vi "About.vi"(0 "path":path) -> ()   [LabVIEW 2013]
uses:
  <vilib>/Platform/browser.llb/Open URL in Default Browser (string).vi
panel:
  out "Author:":string="Martin Šíra"
  out "E-mail:":string="msira@cmi.cz"
  in  "OK":bool
  out "address":string="Czech Metrology Institute\nDepartment of Primary Metrology of\nDC/LF Electrical Quantities\nOkružní 31\n63800, Brno\nCzech Republic"
  out "www:":string="https://qwtb.github.io/qwtb/"
  out "Version:":string
  # "simple QWTB GUI"
  # "Simple QWTB GUI is a front end to a QWTB with graphical user interface.\n\nQWTB is a toolbox for evaluation of measured data. QWTB consist of data processing algorithms from very different sources and unificating application interface. The toolbox gives the possibility to use different data processing algorithms with one set of data and removes the need to reformat data for every particular algorithm. Toolbox is extensible. The toolbox can variate input data and calculate uncertainties by means of Monte Carlo Method (MCM).\n\nToolbox was realized within the EMRP-Project SIB59\nQ-Wave. The EMRP is jointly funded by the EMRP par- ticipating countries within EURAMET and the European Union."
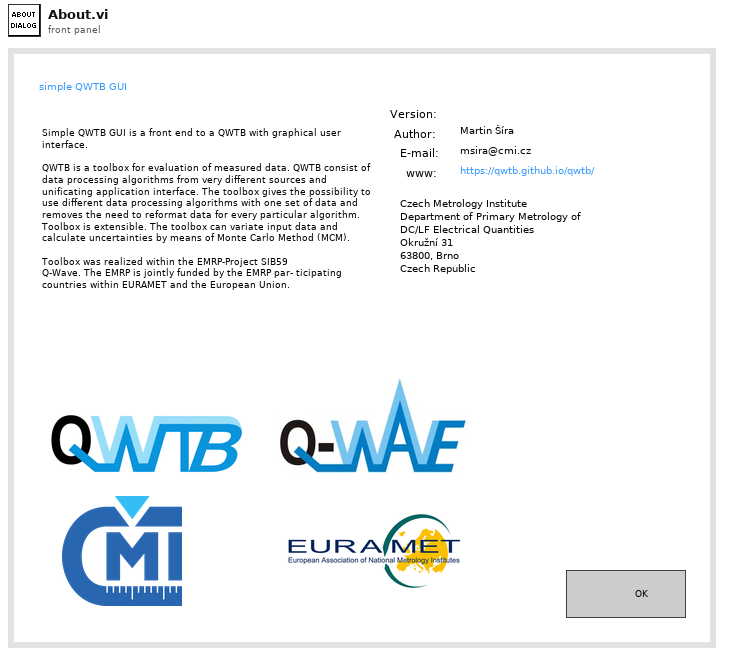
[diagram p1: front panel]
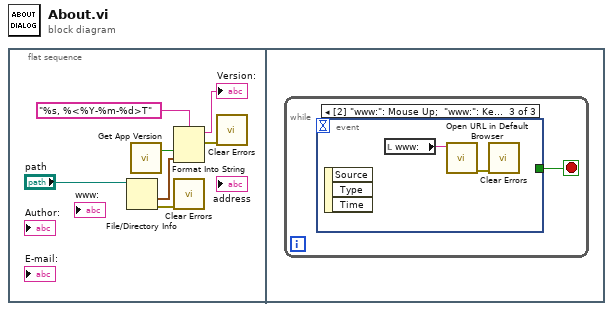
[diagram p0: block diagram]
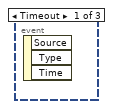
[diagram p2: hidden frame]
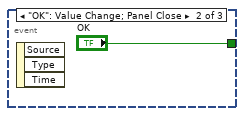
[diagram p3: hidden frame]
diagram:
  n1 = flat-sequence {
    frame #0 {
      n2 = File/Directory Info(path="path") -> (last mod=w4:timestamp, error out=w7:errorcluster)  [unwired: 1 in, 5 out]
      n3 = call "Get App Version.vi"() -> ("runtime"=w3:bool)  [unwired: 1 out]
      n4 = Format Into String(format string="%s, %<%Y-%m-%d>T" ("time format string (%c)"), w3, w4) -> (resulting string=→"Version:":string, error out=w5:errorcluster)  [unwired: 2 in]
      n5 = call <vilib>:"Clear Errors.vi"("error in (no error)"=w7) -> ()  [unwired: 6 in, 1 out]
      n6 = call <vilib>:"Clear Errors.vi"("error in (no error)"=w5) -> ()  [unwired: 6 in, 1 out]
    }
    frame #1 {
      n7 = while {
        stop <- w8 stop-if-true
        n8 = event shown="[2] \"www:\": Mouse Up;  \"www:\": Key Up" {
          selector: _ -> [_ _ _]
          dyn-events: _ -> [_ _ _]
          timeout: _ -> [_ _ _]
          tunnel: [_ "OK" _] -> w8
          event Timeout {
            n9 = event-data() -> ()  [unwired: 1 in, 3 out]
          }
          event "OK": Value Change; Panel Close {
            n10 = event-data() -> ()  [unwired: 1 in, 3 out]
          }
          event "www:": Mouse Up; "www:": Key Up {
            n11 = event-data() -> ()  [unwired: 1 in, 3 out]
            n12 = local read "www:"() -> (w11:string)
            n13 = call-poly <vilib>:"Open URL in Default Browser.vi"("URL"=w11) -> ("error out"=w10:errorcluster)  [unwired: 5 in, 1 out]
            n14 = call <vilib>:"Clear Errors.vi"("error in (no error)"=w10) -> ()  [unwired: 6 in, 1 out]
          }
        }
      }
    }
  }
